vi "UDP Receiver.vi"() -> ()   [LabVIEW 2020]
panel:
  out "data 2":string
  in  "stop 2":bool caption="stop"
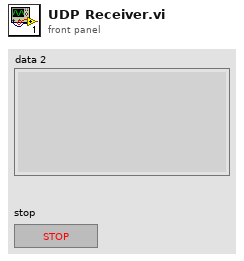
[diagram p1: front panel]
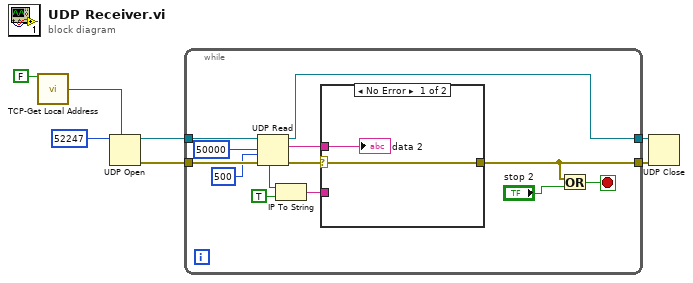
[diagram p0: block diagram]
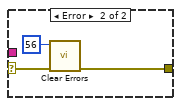
[diagram p2: hidden frame]
diagram:
  n1 = call "TCP-Get Local Address.vi"("LAN first"=FALSE) -> ("net address"=w1:u32)  [unwired: 13 in, 1 out]
  n2 = UDP Open(7:w1, 11:u16 52247 ("port")) -> (port=w6:refnum<k16>, 0:w5:errorcluster)  [unwired: 3 in, 1 out]
  n3 = while {
    tunnel: w6 -> [w20]
    tunnel: w5 -> [w19]
    tunnel: [w14] -> w4
    tunnel: [w17] -> w3
    stop <- w15 stop-if-true
    n4 = UDP Read(connection ID=w20, max size (548)=50000 ("timeout ms (25000)"), timeout ms (25000)=500, 8:w19) -> (data out=w16:string, error out=w18:errorcluster, 3:w17:refnum<k16>, 6:w12:u32)  [unwired: 1 out]
    n5 = IP To String(1:TRUE ("dot notation? (F)"), 2:w12) -> (0:w10:string)
    n6 = case shown="No Error" w18 {
      selector: w18 -> [w21 w25]
      tunnel: [w21 w23] -> w14
      tunnel: w16 -> [w22 _]
      tunnel: w10 -> [_ _]
      frame No Error {
        "data 2" <- w22
      }
      frame Error {
        n7 = call <vilib>:"Clear Errors.vi"("error in (no error)"=w25, "specific error code to clear (0: all)"=56) -> ("error out"=w23:errorcluster)  [unwired: 4 in, 1 out]
      }
    }
    n8 = Or(x=w14, y="stop 2") -> (x .or. y?=w15:bool)
  }
  n9 = UDP Close(connection ID=w3, 8:w4) -> ()  [unwired: 2 out]
